vi "CriticalOpalescenceLogger.vi"() -> ()   [LabVIEW 2014]
uses:
  Typedef_FindPortActions.ctl
  Typedef_TeachLabArduinos.ctl
  Typedef_DataLogger_Actions.ctl
  <vilib>/Utility/file.llb/Write To Spreadsheet File (DBL).vi
panel:
  out "PD vs Time":cluster{dbl[], dbl[]}(graph)
  in  "Time Step (ms)":i32=100 min=5 max=5000 step=1
  out "PD Voltage":dbl format="%.2f"
  out "Fine Temp":string
  out "Coarse Temp":dbl format="%.1f"
  out "PD vs Fine":cluster{dbl[], dbl[]}(graph)
  out "Coarse vs Time":cluster{dbl[], dbl[]}(graph)
  out "Elapsed Time (s)":dbl format="%.1f"
  in  "Filename Header":string="Data"
  in  "Maximum Log Time (s)":dbl=600.0 format="%#_6f"
  out "Status":enum16{"Logging", "Stopped"}(ring)=enum."Stopped"
  in  "Logging":cluster{"Start":bool, "Stop":bool}
  out "Last Save's Filename":string
  in  "Save Data":bool
  in  "Reset Graph":bool
  out "Error Out":errorcluster
  in  "Exit Program":bool
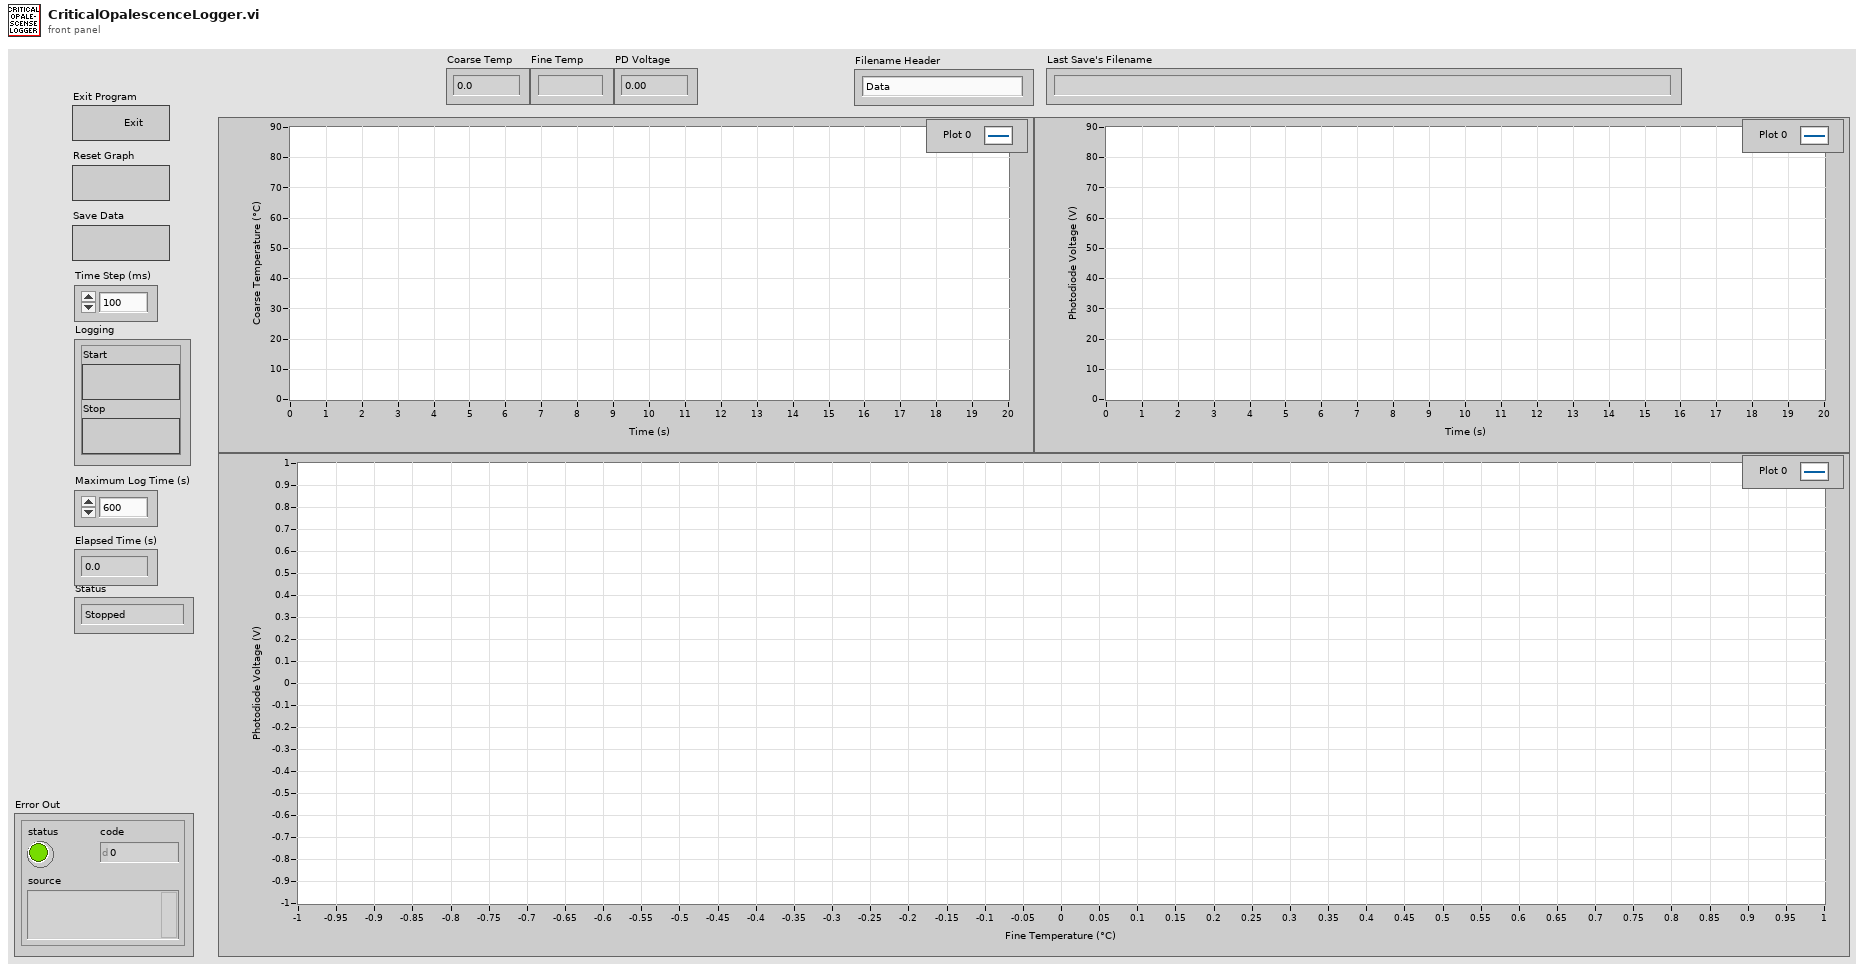
[diagram p1: front panel]
types:
  T1 = typedef "Typedef_FindPortActions.ctl" = enum16{"Reset List", "Find arduinos", "Get COM Port"}
  T2 = typedef "Typedef_TeachLabArduinos.ctl" = enum16{"FH", "AL", "CO", "TD"}
  T3 = typedef "Typedef_DataLogger_Actions.ctl" = enum16{"Connect", "Disconnect", "Get Reading", "Set Offset", "Get Offset", "Set Time Step", "Get Time Step", "Save Settings", "Disable Readings", "Enable Readings"}
  T4 = cluster{cluster{dbl[], dbl[]}, cluster{dbl[], dbl[]}, cluster{dbl[], dbl[]}}
  T5 = cluster{"Coarse Temp":dbl, "Fine Temp":string, "PD Voltage":dbl}
  T6 = cluster{"Course vs Time Out":cluster{"Array":dbl[], "Array":dbl[]}, "PD vs Fine Out":cluster{"Array":dbl[], "Array":dbl[]}, "PD vs Time Out":cluster{"Array":dbl[], "Array":dbl[]}}
  T7 = enum32{"invalid app kind", "Development System", "Run Time System", "Student Edition", "Embedded LabVIEW", "Evaluation", "Custom"}
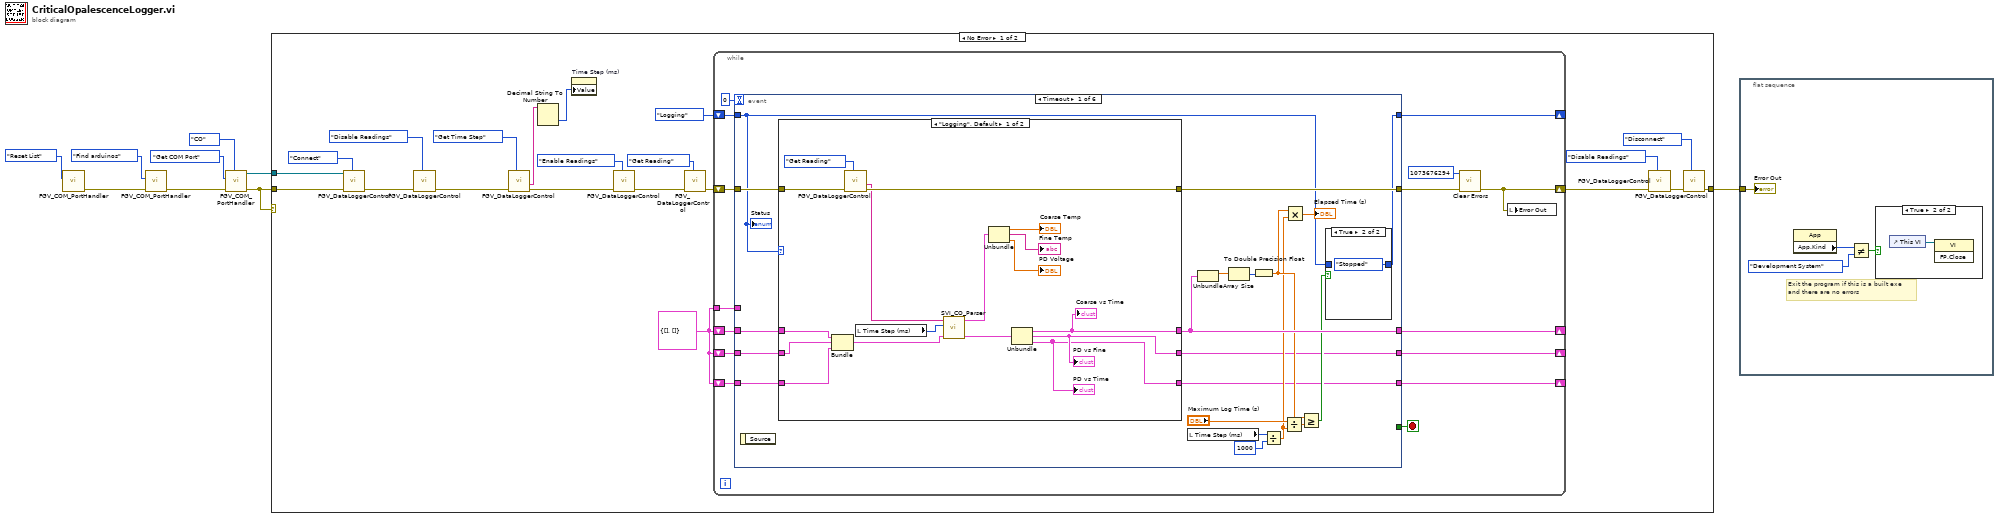
[diagram p0: block diagram]
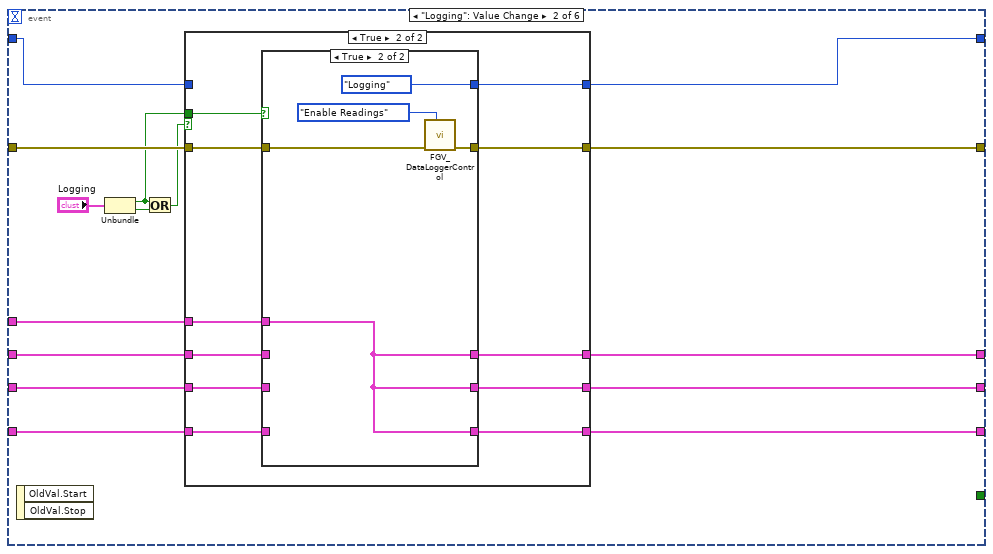
[diagram p5: hidden frame]
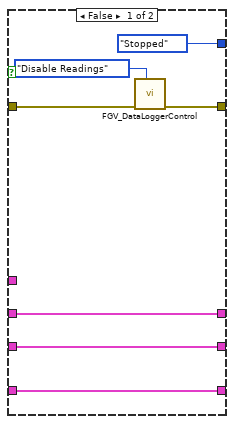
[diagram p7: hidden frame]
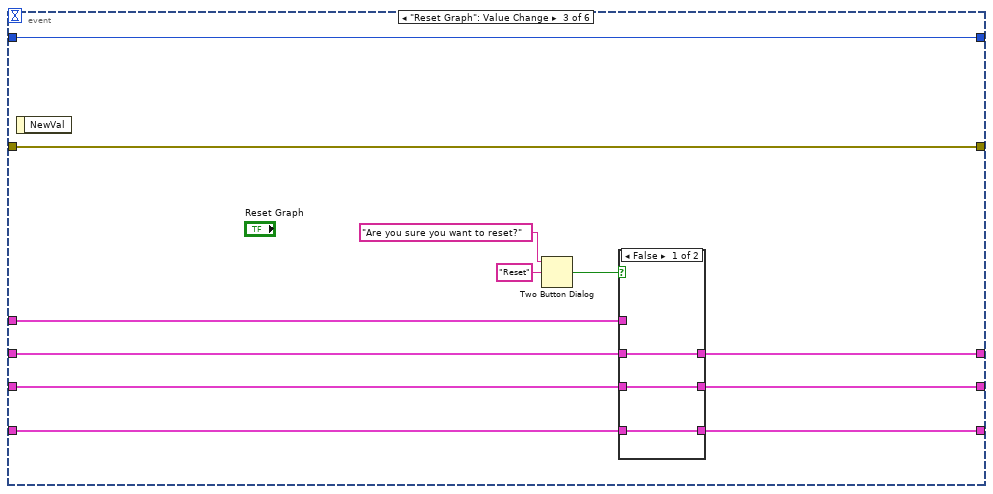
[diagram p8: hidden frame]
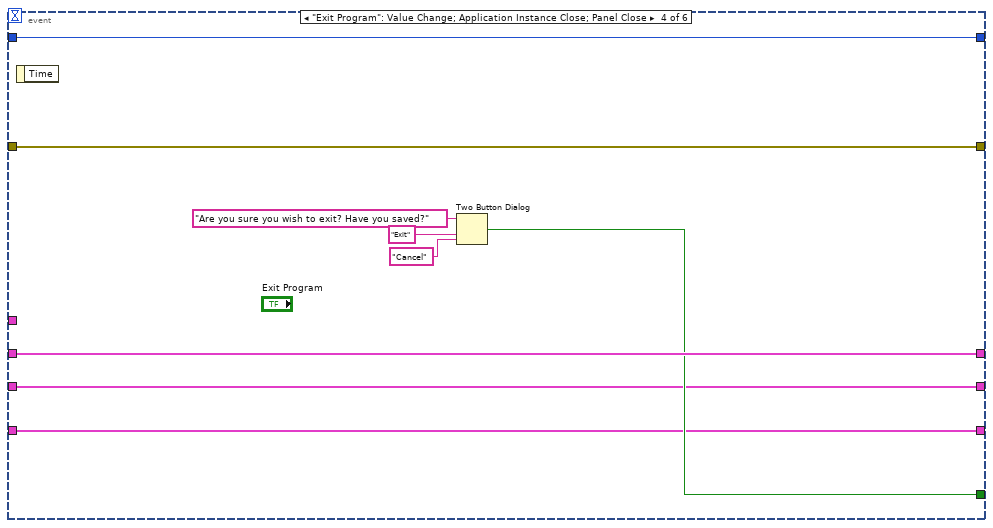
[diagram p10: hidden frame]
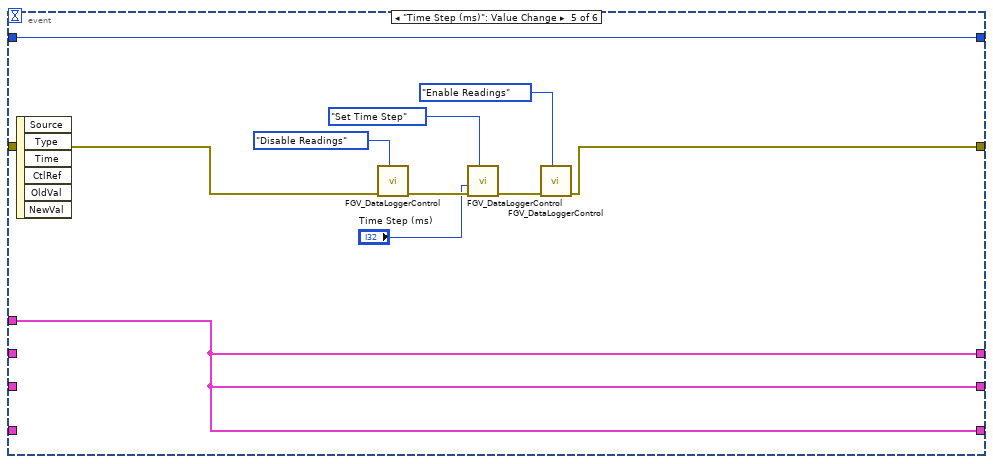
[diagram p11: hidden frame]
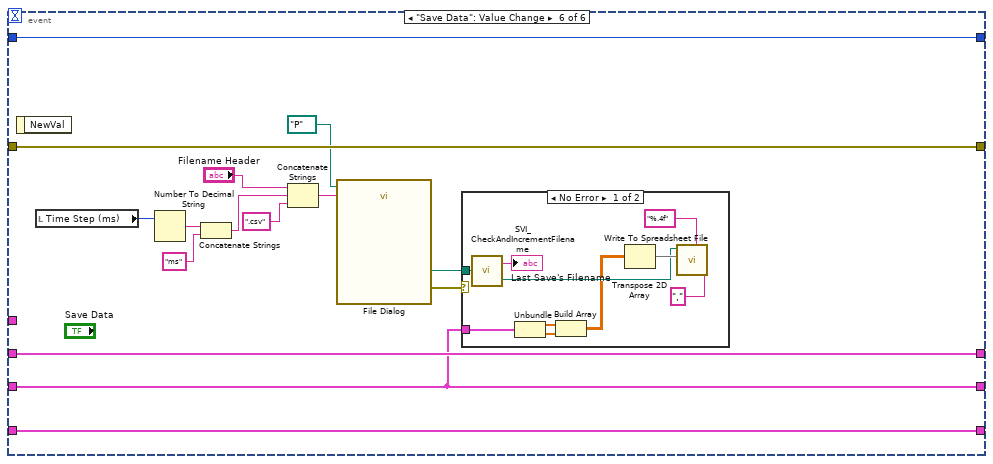
[diagram p12: hidden frame]
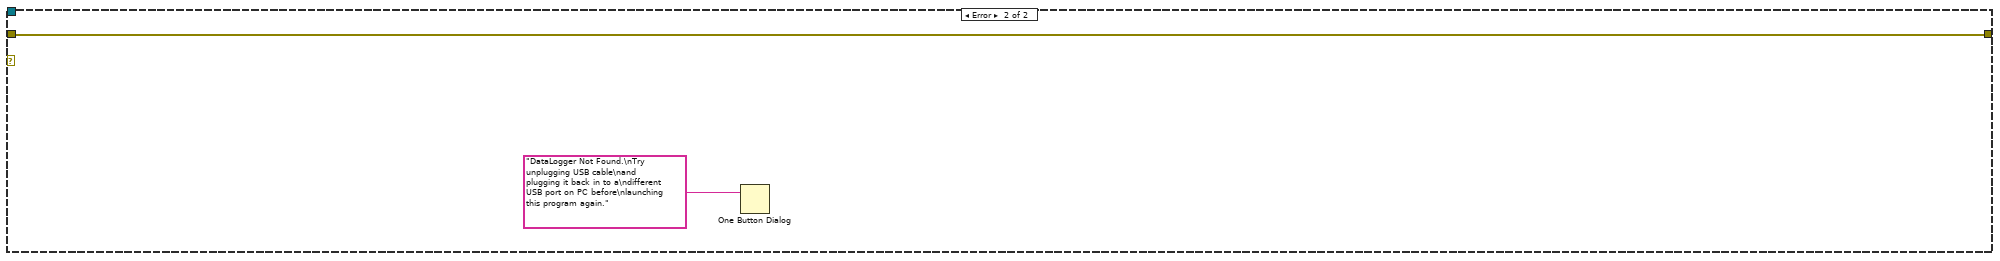
[diagram p14: hidden frame]
diagram:
  n1 = call "FGV_COM_PortHandler.vi"("Action"=Typedef_FindPortActions."Reset List") -> ("Error Out"=w5:errorcluster)  [unwired: 5 in, 2 out]
  n2 = call "FGV_COM_PortHandler.vi"("Error In"=w5, "Action"=Typedef_FindPortActions."Find arduinos") -> ("Error Out"=w9:errorcluster)  [unwired: 4 in, 2 out]
  n3 = call "FGV_COM_PortHandler.vi"("Device"=Typedef_TeachLabArduinos."CO", "Error In"=w9, "Action"=Typedef_FindPortActions."Get COM Port") -> ("Error Out"=w2:errorcluster, "COM Port"=w3:refnum<visa-resource-name>)  [unwired: 3 in, 1 out]
  n4 = case shown="No Error" w2 {
    tunnel: w2 -> [w29 w193]
    tunnel: w3 -> [w28 _]
    tunnel: [w25 w193] -> w1
    frame No Error {
      w10 = cluster{dbl[], dbl[]} {[], []}
      n5 = call "FGV_DataLoggerControl.vi"("Actions"=Typedef_DataLogger_Actions."Connect", "Error In"=w29, "VISA Refnum in"=w28) -> ("Error Out"=w21:errorcluster)  [unwired: 6 in, 2 out]
      n6 = call "FGV_DataLoggerControl.vi"("Actions"=Typedef_DataLogger_Actions."Disable Readings", "Error In"=w21) -> ("Error Out"=w20:errorcluster)  [unwired: 7 in, 2 out]
      n7 = call "FGV_DataLoggerControl.vi"("Actions"=Typedef_DataLogger_Actions."Get Time Step", "Error In"=w20) -> ("Error Out"=w18:errorcluster, "read buffer"=w24:string)  [unwired: 7 in, 1 out]
      n8 = Decimal String To Number(string=w24) -> (number=w23:i32)  [unwired: 2 in, 1 out]
      n9 = property on="Time Step (ms)" class="DigNum (strict)"("Value"=w23) -> ()  [unwired: 2 in, 2 out]
      n10 = call "FGV_DataLoggerControl.vi"("Actions"=Typedef_DataLogger_Actions."Enable Readings", "Error In"=w18) -> ("Error Out"=w11:errorcluster)  [unwired: 7 in, 2 out]
      n11 = call "FGV_DataLoggerControl.vi"("Actions"=Typedef_DataLogger_Actions."Get Reading", "Error In"=w11) -> ("Error Out"=w12:errorcluster)  [unwired: 7 in, 2 out]
      n12 = while {
        shift-right: [w42] -> _
        shift-left: w10 -> [w41]
        tunnel: w10 -> [w40]
        shift-right: [w38] -> _
        shift-left: enum16{"Logging", "Stopped"}."Logging" ("Status") -> [w39]
        shift-right: [w36] -> w16
        shift-left: w12 -> [w45]
        shift-right: [w33] -> _
        shift-left: w10 -> [w34]
        shift-right: [w31] -> _
        shift-left: w10 -> [w32]
        stop <- w44 stop-if-true
        n13 = event shown="[0] Timeout" {
          selector: _ -> [_ _ _ _ _ _]
          dyn-events: _ -> [_ _ _ _ _ _]
          timeout: 0 -> [_ _ _ _ _ _]
          tunnel: w45 -> [w65 w101 w143 w155 w160 w181]
          tunnel: [w64 w100 w143 w155 w161 w181] -> w35
          tunnel: [_ _ _ w151 _ _] -> w44
          tunnel: [w61 w94 w137 w156 w158 w180] -> w42
          tunnel: w41 -> [w63 w95 w134 w156 _ w180]
          tunnel: w40 -> [_ w93 w138 _ w158 _]
          tunnel: [w54 w103 w142 w150 w159 w172] -> w38
          tunnel: w39 -> [w53 w102 w142 w150 w159 w172]
          tunnel: w34 -> [w49 w91 w133 w149 _ w170]
          tunnel: [w48 w92 w136 w149 w158 w170] -> w33
          tunnel: w32 -> [w47 w90 w132 w148 _ w169]
          tunnel: [w46 w89 w135 w148 w158 w169] -> w31
          event Timeout {
            n14 = event-data() -> ()  [unwired: 1 in, 1 out]
            n15 = case shown="\"Logging\", Default" w53 {
              tunnel: w65 -> [w84 w87]
              tunnel: [w83 w87] -> w64
              tunnel: [w70 w88] -> w61
              tunnel: w63 -> [w78 w88]
              tunnel: w49 -> [w77 w86]
              tunnel: [w69 w86] -> w48
              tunnel: w47 -> [w71 w85]
              tunnel: [w68 w85] -> w46
              frame "Logging", Default {
                n16 = Bundle(w78, w77, w71) -> (w79:T4)  [unwired: 1 in]
                n17 = call "FGV_DataLoggerControl.vi"("Actions"=Typedef_DataLogger_Actions."Get Reading", "Error In"=w84) -> ("Error Out"=w83:errorcluster, "read buffer"=w81:string)  [unwired: 7 in, 1 out]
                n18 = local read "Time Step (ms)"() -> (w73:i32)
                n19 = call "SVI_CO_Parser.vi"("read buffer"=w81, "Time Step (ms)"=w73, "In"=w79) -> ("Current Values"=w72:T5, "Out"=w80:T6)  [unwired: 4 in]
                n20 = Unbundle(w72) -> ("Coarse Temp"=→"Coarse Temp":dbl, "Fine Temp"=→"Fine Temp":string, "PD Voltage"=→"PD Voltage":dbl)
                n21 = Unbundle(w80) -> ("Course vs Time Out"=w70:cluster{"Array":dbl[], "Array":dbl[]}, "PD vs Fine Out"=w69:cluster{"Array":dbl[], "Array":dbl[]}, "PD vs Time Out"=w68:cluster{"Array":dbl[], "Array":dbl[]})
                "PD vs Fine" <- w69
                "Coarse vs Time" <- w70
                "PD vs Time" <- w68
              }
              frame "Stopped" {
              }
            }
            n22 = local read "Time Step (ms)"() -> (w60:i32)
            n23 = Unbundle(w61) -> ("Array"=w62:dbl[])  [unwired: 1 out]
            n24 = Array Size(array=w62) -> (size(s)=w56:i32)
            n25 = To Double Precision Float(number=w56) -> (double precision float=w52:dbl)
            n26 = Divide(x=w60, y=1000) -> (x/y=w51:dbl)
            n27 = Divide(x="Maximum Log Time (s)", y=w51) -> (x/y=w57:dbl)
            n28 = Multiply(x=w52, y=w51) -> (x*y=→"Elapsed Time (s)":dbl)
            n29 = Greater Or Equal?(x=w52, y=w57) -> (x >= y?=w55:bool)
            n30 = case shown="True" w55 {
              tunnel: [w66 enum16{"Logging", "Stopped"}."Stopped" ("Status")] -> w54
              tunnel: w53 -> [w66 _]
              frame False {
              }
              frame True {
              }
            }
            "Status" <- w53
          }
          event "Logging": Value Change {
            n31 = event-data() -> ()  [unwired: 1 in, 2 out]
            n32 = Unbundle("Logging") -> ("Start"=w96:bool, "Stop"=w98:bool)
            n33 = Or(x=w96, y=w98) -> (x .or. y?=w97:bool)
            n34 = case shown="True" w97 {
              tunnel: [w108 w119] -> w103
              tunnel: w102 -> [w108 _]
              tunnel: w101 -> [w107 w118]
              tunnel: [w107 w117] -> w100
              tunnel: w96 -> [_ w116]
              tunnel: w95 -> [w106 w115]
              tunnel: [w106 w114] -> w94
              tunnel: w93 -> [_ w113]
              tunnel: [w105 w112] -> w92
              tunnel: w91 -> [w105 w111]
              tunnel: w90 -> [w104 w110]
              tunnel: [w104 w109] -> w89
              frame False {
              }
              frame True {
                n35 = case shown="True" w116 {
                  tunnel: [enum16{"Logging", "Stopped"}."Stopped" ("Status") enum16{"Logging", "Stopped"}."Logging" ("Status")] -> w119
                  tunnel: w118 -> [w123 w129]
                  tunnel: [w124 w128] -> w117
                  tunnel: w115 -> [w122 _]
                  tunnel: [w122 w127] -> w114
                  tunnel: w113 -> [_ w127]
                  tunnel: [w121 w127] -> w112
                  tunnel: w111 -> [w121 _]
                  tunnel: w110 -> [w120 _]
                  tunnel: [w120 w127] -> w109
                  frame False {
                    n36 = call "FGV_DataLoggerControl.vi"("Actions"=Typedef_DataLogger_Actions."Disable Readings", "Error In"=w123) -> ("Error Out"=w124:errorcluster)  [unwired: 7 in, 2 out]
                  }
                  frame True {
                    n37 = call "FGV_DataLoggerControl.vi"("Actions"=Typedef_DataLogger_Actions."Enable Readings", "Error In"=w129) -> ("Error Out"=w128:errorcluster)  [unwired: 7 in, 2 out]
                  }
                }
              }
            }
          }
          event "Reset Graph": Value Change {
            n38 = event-data() -> ()  [unwired: 1 in, 1 out]
            n39 = Two Button Dialog(message="Are you sure you want to reset?", 2:"Reset" ("T button name (\"OK\")")) -> (T button?=w139:bool)  [unwired: 1 in]
            n40 = case shown="False" w139 {
              tunnel: w138 -> [_ w147]
              tunnel: [w146 w147] -> w137
              tunnel: [w145 w147] -> w136
              tunnel: [w144 w147] -> w135
              tunnel: w134 -> [w146 _]
              tunnel: w133 -> [w145 _]
              tunnel: w132 -> [w144 _]
              frame False {
              }
              frame True {
              }
            }
          }
          event "Exit Program": Value Change; Application Instance Close; Panel Close {
            n41 = event-data() -> ()  [unwired: 1 in, 1 out]
            n42 = Two Button Dialog(message="Are you sure you wish to exit? Have you saved?", 1:"Cancel" ("F button name (\"Cancel\")"), 2:"Exit" ("T button name (\"OK\")")) -> (T button?=w151:bool)
          }
          event "Time Step (ms)": Value Change {
            n43 = event-data() -> ()  [unwired: 1 in, 6 out]
            n44 = call "FGV_DataLoggerControl.vi"("Actions"=Typedef_DataLogger_Actions."Disable Readings", "Error In"=w160) -> ("Error Out"=w164:errorcluster)  [unwired: 7 in, 2 out]
            n45 = call "FGV_DataLoggerControl.vi"("Actions"=Typedef_DataLogger_Actions."Set Time Step", "Error In"=w164, "Value"="Time Step (ms)") -> ("Error Out"=w162:errorcluster)  [unwired: 6 in, 2 out]
            n46 = call "FGV_DataLoggerControl.vi"("Actions"=Typedef_DataLogger_Actions."Enable Readings", "Error In"=w162) -> ("Error Out"=w161:errorcluster)  [unwired: 7 in, 2 out]
          }
          event "Save Data": Value Change {
            n47 = event-data() -> ()  [unwired: 1 in, 1 out]
            n48 = local read "Time Step (ms)"() -> (w173:i32)
            n49 = Number To Decimal String(number=w173) -> (decimal integer string=w174:string)  [unwired: 1 in]
            n50 = Concatenate Strings(w174, "ms" ("string")) -> (w176:string)
            n51 = Concatenate Strings("Filename Header", w176, ".csv" ("default name")) -> (w178:string)
            n52 = call "File Dialog"("start path"=path "P:/", "default name"=w178) -> ("selected path"=w179:path, "error out"=w167:errorcluster)  [unwired: 10 in, 2 out]
            n53 = case shown="No Error" w167 {
              tunnel: w179 -> [w188 _]
              tunnel: w170 -> [w182 _]
              frame No Error {
                n54 = call "SVI_CheckAndIncrementFilename.vi"("selected path"=w188) -> ("Filename"=→"Last Save's Filename":string, "File Path"=w185:path)
                n55 = Unbundle(w182) -> (w190:dbl[], w191:dbl[])
                n56 = Build Array(w190, w191) -> (w184:dbl[][])
                n57 = Transpose 2D Array(2D array=w184) -> (transposed array=w186:dbl[][])
                n58 = call-poly <vilib>:"Write To Spreadsheet File.vi"("delimiter (\\t)"="," ("delimiter (\\t)"), "format (%.3f)"="%.4f", "2D data"=w186, "file path (dialog if empty)"=w185) -> ()  [unwired: 4 in, 1 out]
              }
              frame Error {
              }
            }
          }
        }
        n59 = call <vilib>:"Clear Errors.vi"("error in (no error)"=w35, "specific error code to clear (0: all)"=1073676294) -> ("error out"=w36:errorcluster)  [unwired: 4 in, 1 out]
        n60 = local write "Error Out"(w36) -> ()
      }
      n61 = call "FGV_DataLoggerControl.vi"("Actions"=Typedef_DataLogger_Actions."Disable Readings", "Error In"=w16) -> ("Error Out"=w15:errorcluster)  [unwired: 7 in, 2 out]
      n62 = call "FGV_DataLoggerControl.vi"("Actions"=Typedef_DataLogger_Actions."Disconnect", "Error In"=w15) -> ("Error Out"=w25:errorcluster)  [unwired: 7 in, 2 out]
    }
    frame Error {
      n63 = One Button Dialog(message="DataLogger Not Found.\nTry unplugging USB cable\nand plugging it back in to a\ndifferent USB port on PC before\nlaunching this program again.") -> ()  [unwired: 1 in, 1 out]
    }
  }
  n64 = flat-sequence {
    tunnel: w1 -> [w195]
    frame #0 {
      # "Exit the program if this is a built exe\nand there are no errors"
      n65 = property class="App"() -> ("App.Kind"=w196:T7)  [unwired: 2 in, 2 out]
      n66 = Not Equal?(x=w196, y=T7."Development System" ("Application:Kind 2")) -> (x != y?=w194:bool)
      n67 = case shown="True" w194 {
        frame False {
        }
        frame True {
          n68 = control-ref of="This VI"() -> (w198:refnum<vi>)
          n69 = invoke class="VI" method="FP.Close"(reference=w198) -> ()  [unwired: 2 in, 3 out]
        }
      }
      "Error Out" <- w195
    }
  }
